vi "Get message from save image VI.vi"(8 "error in (no error)":errorcluster, 11 "Channel in":refnum<class "Channel.lvclass">) -> (0 "error out":errorcluster, 3 "Channel out":refnum<class "Channel.lvclass">)   [LabVIEW 2018, in "Channel.lvclass"]
doc: "Get message from the save image VI"
uses:
  Channel.lvclass
  Channel.lvclass/Channel.ctl
  RxTx/RxTx.lvclass
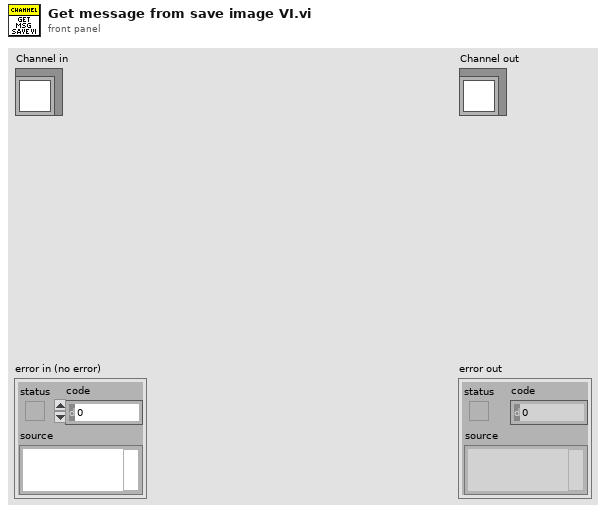
[diagram p1: front panel]
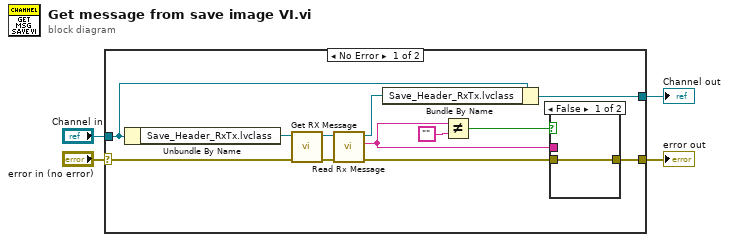
[diagram p0: block diagram]
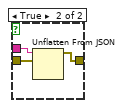
[diagram p2: hidden frame]
diagram:
  n1 = case shown="No Error" "error in (no error)" {
    selector: "error in (no error)" -> [w11 w22]
    tunnel: [w5 w22] -> w3
    tunnel: [w15 w21] -> w1
    tunnel: "Channel in" -> [w16 w21]
    frame No Error {
      n2 = Unbundle By Name(w16) -> ("Save_Header_RxTx.lvclass"=w14:refnum<class "RxTx.lvclass">)
      n3 = call "Get RX Message.vi"("error in (no error)"=w11, "RxTx in"=w14) -> ("error out"=w10:errorcluster, "RxTx out"=w13:refnum<class "RxTx.lvclass">)  [unwired: 8 in]
      n4 = call "Read Rx Message.vi"("error in (no error)"=w10, "RxTx in"=w13) -> ("error out"=w6:errorcluster, "Rx Message"=w9:string, "RxTx out"=w12:refnum<class "RxTx.lvclass">)  [unwired: 7 in]
      n5 = Bundle By Name(cluster=w16, "Save_Header_RxTx.lvclass"=w12) -> (w15:refnum<class "Channel.lvclass">)
      n6 = Not Equal?(x=w9, y="") -> (x != y?=w8:bool)
      n7 = case shown="False" w8 {
        tunnel: w6 -> [w17 w20]
        tunnel: w9 -> [_ w19]
        tunnel: [w17 w18] -> w5
        frame False {
        }
        frame True {
          n8 = Unflatten From JSON(JSON string=w19, type and defaults=w20) -> (value=w18:errorcluster)  [unwired: 5 in, 1 out]
        }
      }
    }
    frame Error {
    }
  }
  "error out" <- w3
  "Channel out" <- w1
